vi "全局变量.vi"() -> ()   [LabVIEW 2018]
panel:
  in  "实验标识符":string
  in  "枚举值":i8
  in  "串口":refnum<visa-resource-name>
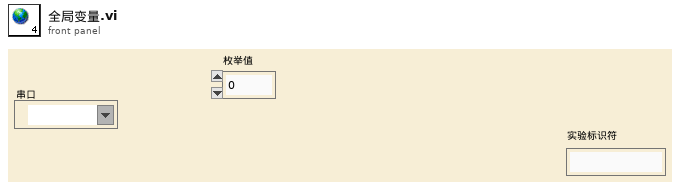
[diagram p1: front panel]
diagram:
